vi "myRIO_BRig_RT__Case_NonExp_State_DispenseWater.vi"(9 "input_increment":i64, 10 "input_state":T1, 11 "input_dataMTrig":u16[](array[numeric])) -> (0 "output_dispense__R":bool, 1 "output_dispense__L":bool, 2 "output_state":T1, 3 "output_dataMTrig":u16[](array[numeric]))   [LabVIEW 2014]
uses:
  myRIO_Gil_RT__stateList_7,4__NoExp.ctl
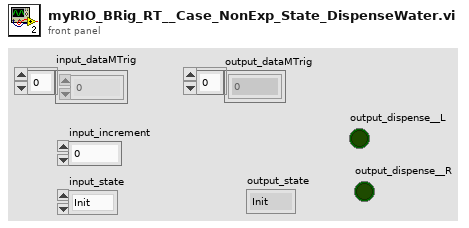
[diagram p1: front panel]
types:
  T1 = typedef "myRIO_Gil_RT__stateList_7,4__NoExp.ctl" = enum16{"Init", "UploadSettings", "Idle", "RewardCalibration_pre", "DispenseWater_pre", "DispenseWater", "DispenseWater_Delay_pre", "DispenseWater_Delay", "TestConnection", "End"}
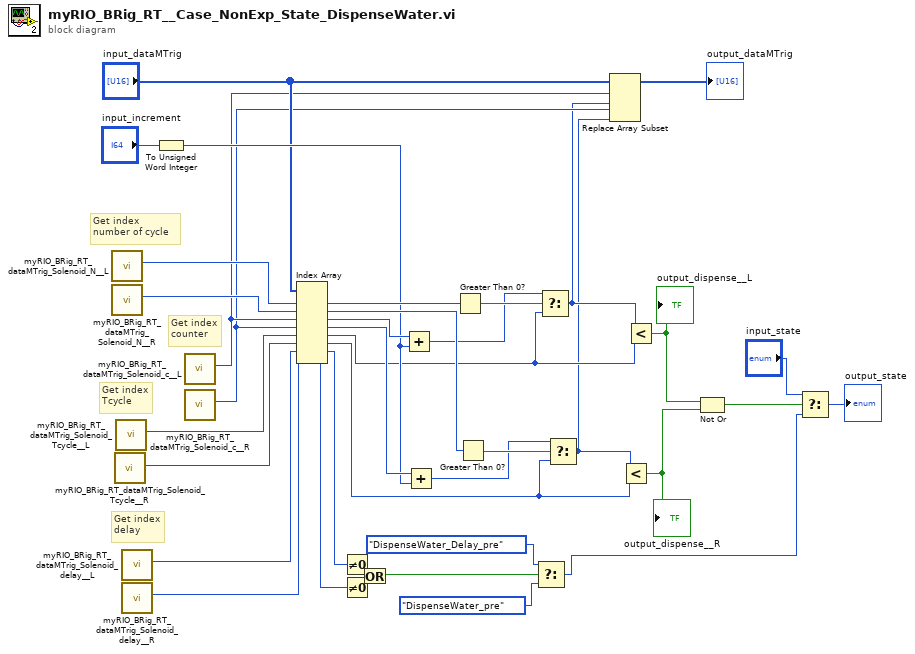
[diagram p0: block diagram]
diagram:
  # "Get index\ndelay"
  # "Get index\nTcycle"
  # "Get index\nnumber of cycle"
  # "Get index\ncounter"
  n1 = call "myRIO_BRig_RT_dataMTrig_Solenoid_N__L.vi"() -> ("output_Solenoid_N__L"=w37:i32)  [unwired: 11 in]
  n2 = call "myRIO_BRig_RT_dataMTrig_Solenoid_N__R.vi"() -> ("output_Solenoid_N__R"=w36:i32)  [unwired: 11 in]
  n3 = call "myRIO_BRig_RT_dataMTrig_Solenoid_Tcycle__R.vi"() -> ("output_Solenoid_Tcycle__R"=w34:i32)  [unwired: 11 in]
  n4 = call "myRIO_BRig_RT_dataMTrig_Solenoid_Tcycle__L.vi"() -> ("output_Solenoid_Tcycle__L"=w35:i32)  [unwired: 11 in]
  n5 = call "myRIO_BRig_RT_dataMTrig_Solenoid_delay__L.vi"() -> ("output_Solenoid_delay__L"=w13:i32)  [unwired: 11 in]
  n6 = call "myRIO_BRig_RT_dataMTrig_Solenoid_delay__R.vi"() -> ("output_Solenoid_delay__R"=w12:i32)  [unwired: 11 in]
  n7 = To Unsigned Word Integer(number="input_increment") -> (unsigned 16bit integer=w28:u16)
  n8 = call "myRIO_BRig_RT_dataMTrig_Solenoid_c__L.vi"() -> ("output_Solenoid_c__L"=w19:i32)  [unwired: 11 in]
  n9 = call "myRIO_BRig_RT_dataMTrig_Solenoid_c__R.vi"() -> ("output_Solenoid_c__R"=w18:i32)  [unwired: 11 in]
  n10 = Index Array(array="input_dataMTrig", index #1=w37, index #2=w36, index #3=w19, index #4=w18, index #5=w35, index #6=w34, index #7=w13, index #8=w12) -> (element #1=w33:u16, element #2=w32:u16, element #3=w30:u16, element #4=w29:u16, element #5=w23:u16, element #6=w22:u16, element #7=w9:u16, element #8=w8:u16)
  n11 = Not Equal To 0?(x=w9) -> (x != 0?=w10:bool)
  n12 = Not Equal To 0?(x=w8) -> (x != 0?=w11:bool)
  n13 = Or(x=w10, y=w11) -> (x .or. y?=w6:bool)
  n14 = Add(x=w30, y=w28) -> (x+y=w26:u16)
  n15 = Add(x=w29, y=w28) -> (x+y=w24:u16)
  n16 = Greater Than 0?(x=w33) -> (x > 0?=w27:bool)
  n17 = Greater Than 0?(x=w32) -> (x > 0?=w25:bool)
  n18 = Select(t=myRIO_Gil_RT__stateList_7,4__NoExp."DispenseWater_Delay_pre", s=w6, f=myRIO_Gil_RT__stateList_7,4__NoExp."DispenseWater_pre" ("t")) -> (s? t:f=w3:T1)
  n19 = Select(t=w26, s=w27, f=w23) -> (s? t:f=w17:u16)
  n20 = Select(t=w24, s=w25, f=w22) -> (s? t:f=w16:u16)
  n21 = Replace Array Subset(array="input_dataMTrig", new element #1=w17, index #1=w19, new element #2=w16, index #2=w18) -> (→"output_dataMTrig":u16[])
  n22 = Less?(x=w16, y=w22) -> (x < y?=w14:bool)
  "output_dispense__R" <- w14
  n23 = Less?(x=w17, y=w23) -> (x < y?=w15:bool)
  "output_dispense__L" <- w15
  n24 = Not Or(1:w14, 2:w15) -> (0:w7:bool)
  n25 = Select(t="input_state", s=w7, f=w3) -> (s? t:f=→"output_state":T1)
